vi "SeqnPool.vi"() -> ()   [LabVIEW 2012, in "StimulCtrls.lvlib"]
uses:
  StimulCtrls.lvlib
  UserControl/Cohort_sm.ctl
  UserControl/ElectdTerminal.ctl
  Sequence.lvclass
  Cohort.lvclass
panel:
  out "Seqn out":refnum<class "Sequence.lvclass">[](array[class])
  in  "Seqn in":refnum<class "Sequence.lvclass">[](array[class])
  in  "Pool":T3
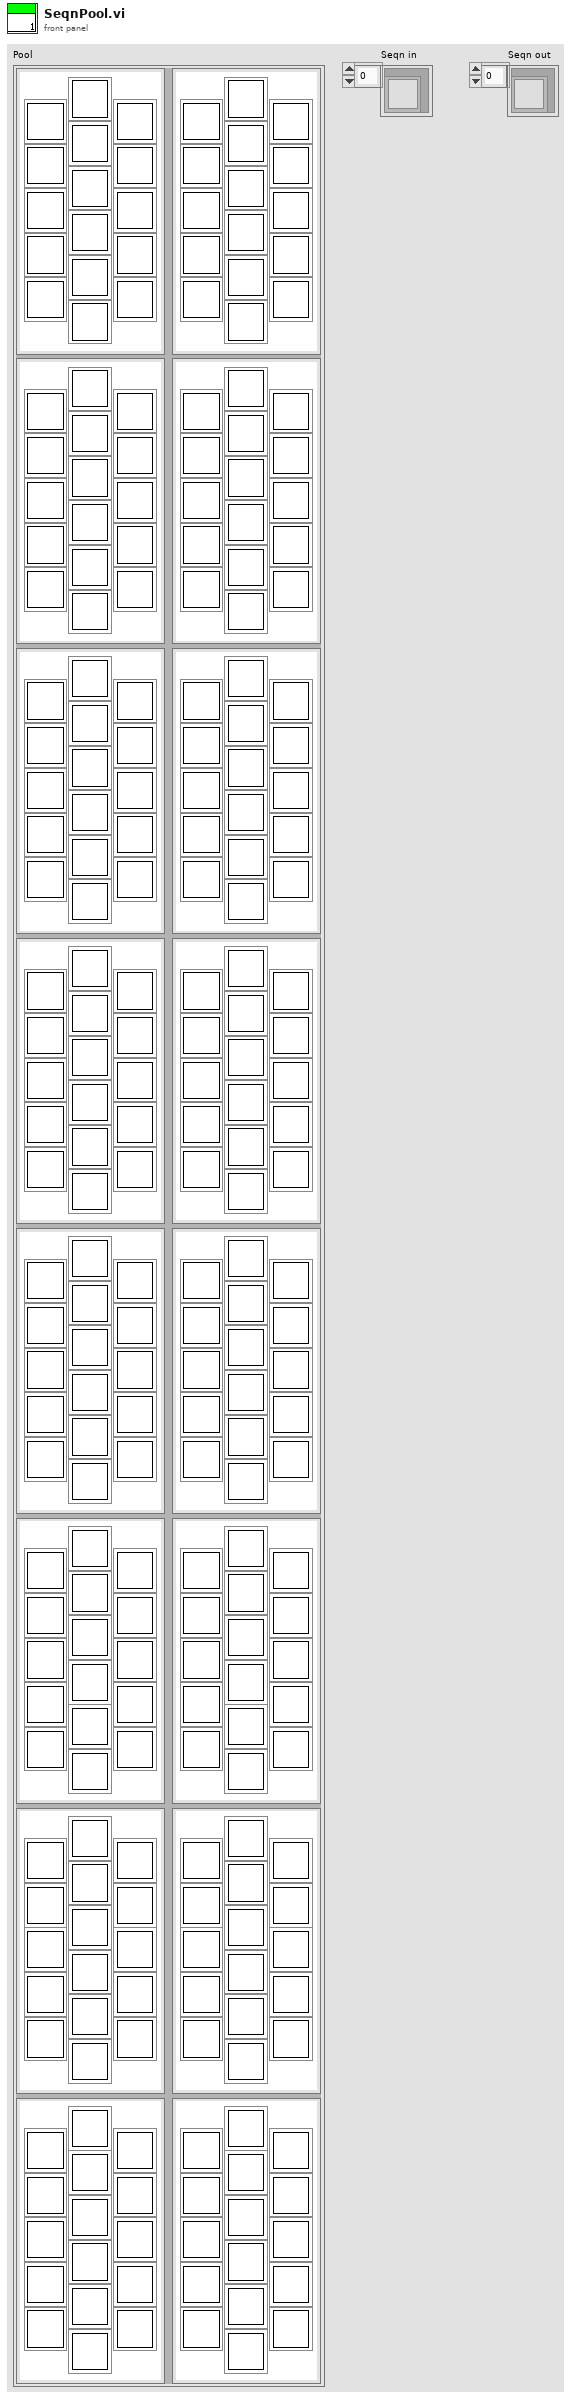
[diagram p1: front panel]
types:
  T1 = typedef "StimulCtrls.lvlib/Cohort_sm.ctl" = cluster{"T 5":T2, "T 6":T2, "T 7":T2, "T 8":T2, "T 9":T2, "T 10":T2, "T 11":T2, "T 12":T2, "T 13":T2, "T 14":T2, "T 15":T2, "T 0":T2, "T 1":T2, "T 2":T2, "T 3":T2, "T 4":T2}
  T2 = typedef "StimulCtrls.lvlib/ElectdTerminal.ctl" = u8
  T3 = cluster{"Seed 0":T1, "Seed 1":T1, "Seed 2":T1, "Seed 3":T1, "Seed 4":T1, "Seed 5":T1, "Seed 6":T1, "Seed 7":T1, "Seed 8":T1, "Seed 9":T1, "Seed 10":T1, "Seed 11":T1, "Seed 12":T1, "Seed 13":T1, "Seed 14":T1, "Seed 15":T1}
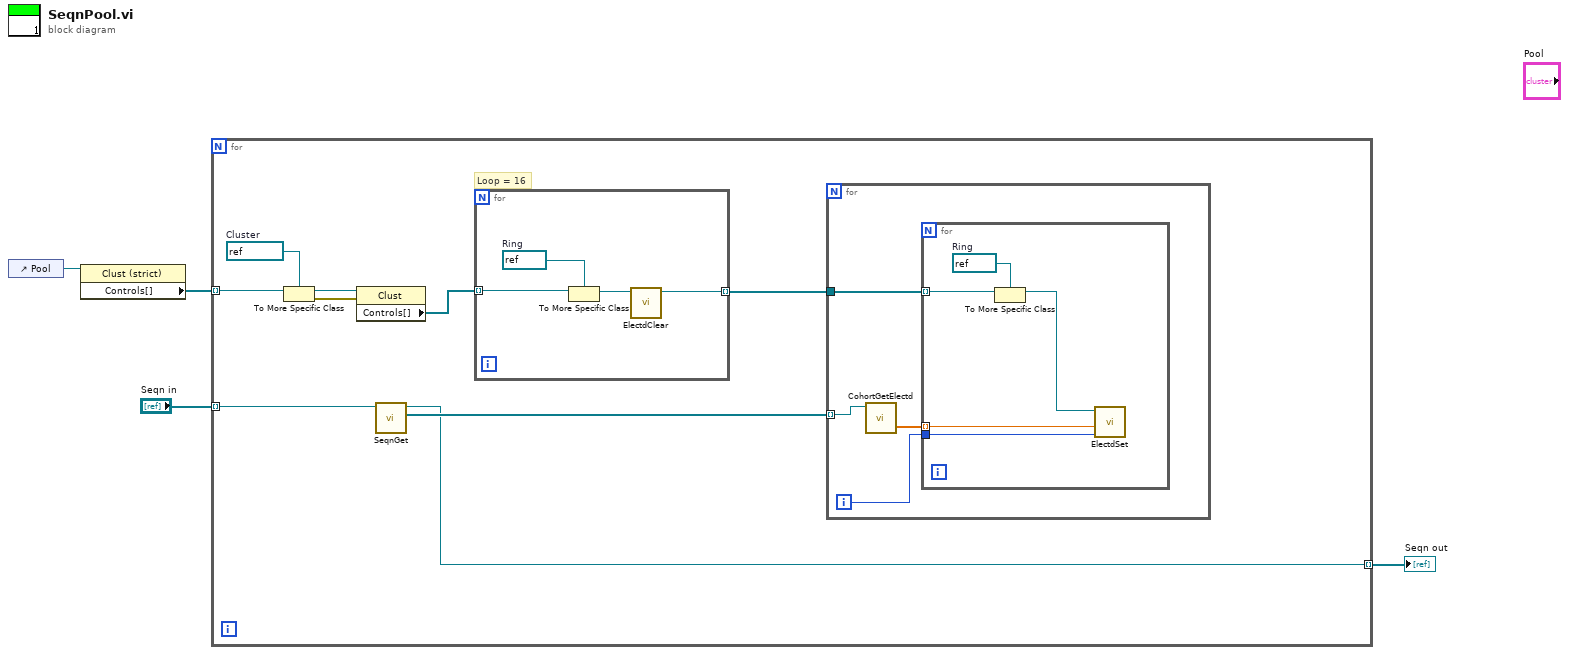
[diagram p0: block diagram]
diagram:
  n1 = control-ref of="Pool"() -> (w4:refnum<vi>)
  n2 = property class="Clust (strict)"(reference=w4) -> ("Controls[]"=w3:refnum<vi>[])  [unwired: 1 in, 2 out]
  n3 = for {
    tunnel: "Seqn in" -> [w8] mode=indexing
    tunnel: w3 -> [w13] mode=indexing
    tunnel: [w5] -> w1 mode=indexing
    w12 = refnum<vi> refnum  # Cluster
    # "Loop = 16"
    n4 = To More Specific Class(target class=w12, reference=w13) -> (specific class reference=w11:refnum<vi>, error out=w10:errorcluster)  [unwired: 1 in]
    n5 = property class="Clust"(reference=w11, error in=w10) -> ("Controls[]"=w9:refnum<vi>[])  [unwired: 2 out]
    n6 = call-dynamic "SeqnGet.vi"("Sequence in"=w8) -> ("Cohorts"=w6:refnum<class "Cohort.lvclass">[], "Sequence out"=w5:refnum<class "Sequence.lvclass">)  [unwired: 8 in, 1 out]
    n7 = for {
      tunnel: w9 -> [w26] mode=indexing
      tunnel: [w23] -> w7 mode=indexing
      w25 = refnum<vi> refnum  # Ring
      n8 = To More Specific Class(target class=w25, reference=w26) -> (specific class reference=w24:refnum<vi>)  [unwired: 1 in, 1 out]
      n9 = call "ElectdClear.vi"("Electd in"=w24) -> ("Electd out"=w23:refnum<vi>)  [unwired: 10 in]
    }
    n10 = for {
      tunnel: w6 -> [w17] mode=indexing
      tunnel: w7 -> [w15]
      i -> [w14]
      n11 = call-dynamic "CohortGetElectd.vi"("Cohort in"=w17) -> ("Amplitude"=w16:sgl[])  [unwired: 6 in, 4 out]
      n12 = for {
        tunnel: w16 -> [w22] mode=indexing
        tunnel: w15 -> [w20] mode=indexing
        tunnel: w14 -> [w18]
        w21 = refnum<vi> refnum  # Ring
        n13 = To More Specific Class(target class=w21, reference=w20) -> (specific class reference=w19:refnum<vi>)  [unwired: 1 in, 1 out]
        n14 = call "ElectdSet.vi"("Group #"=w18, "Amplitude"=w22, "Electd Panel in"=w19) -> ()  [unwired: 8 in, 1 out]
      }
    }
  }
  "Seqn out" <- w1
